vi "Get Data Type Prefix.vi"(3 "Data type":T2) -> (0 "data type":T1="double precision", 1 "data type prefix":string)   [LabVIEW 2019, in "LV-Data.PGSQL.lvclass"]
uses:
  LV-Data.PGSQL.lvclass
  Typedefs/Datatypes--enum.ctl
  Typedefs/Datatypes--combo.ctl
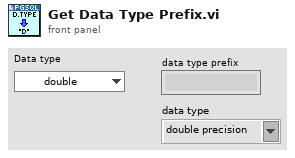
[diagram p1: front panel]
types:
  T1 = typedef "LV-Data.PGSQL.lvclass/Datatypes--combo.ctl" = string
  T2 = typedef "LV-Data.PGSQL.lvclass/Datatypes--enum.ctl" = enum16{"double", "string", "json", "integer", "boolean"}
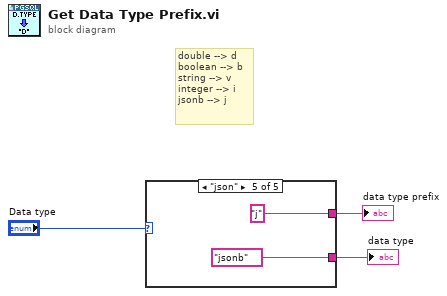
[diagram p0: block diagram]
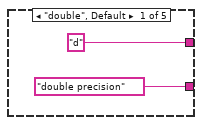
[diagram p2: hidden frame]
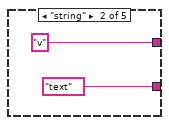
[diagram p3: hidden frame]
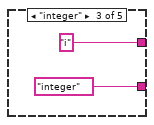
[diagram p4: hidden frame]
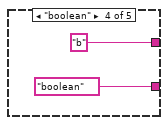
[diagram p5: hidden frame]
diagram:
  # "double --> d\nboolean --> b\nstring --> v\ninteger --> i\njsonb --> j"
  n1 = case shown="\"json\"" "Data type" {
    tunnel: ["d" "v" "i" "b" "j"] -> w2
    tunnel: [T1 "double precision" ("new column data type") T1 "text" ("new column data type") T1 "integer" ("new column data type") T1 "boolean" ("new column data type") T1 "jsonb" ("new column data type")] -> w1
    frame "double", Default {
    }
    frame "string" {
    }
    frame "integer" {
    }
    frame "boolean" {
    }
    frame "json" {
    }
  }
  "data type prefix" <- w2
  "data type" <- w1
